vi "Configure Results Names.vi"(8 "error in":errorcluster, 11 "DAC ADV in":refnum<class "DAC ADV.lvclass">) -> (0 "error out":errorcluster, 3 "DAC ADV out":refnum<class "DAC ADV.lvclass">)   [LabVIEW 2019, in "DAC.lvlib" / "DAC ADV.lvclass"]
uses:
  DAC ADV.lvclass
  DAC ADV.lvclass/DAC ADV.ctl
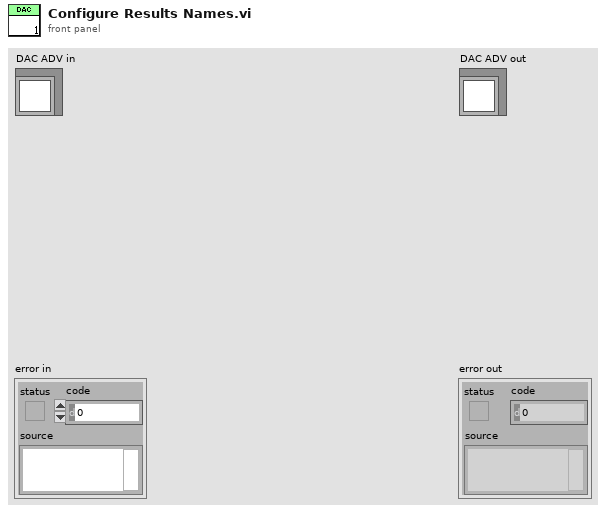
[diagram p1: front panel]
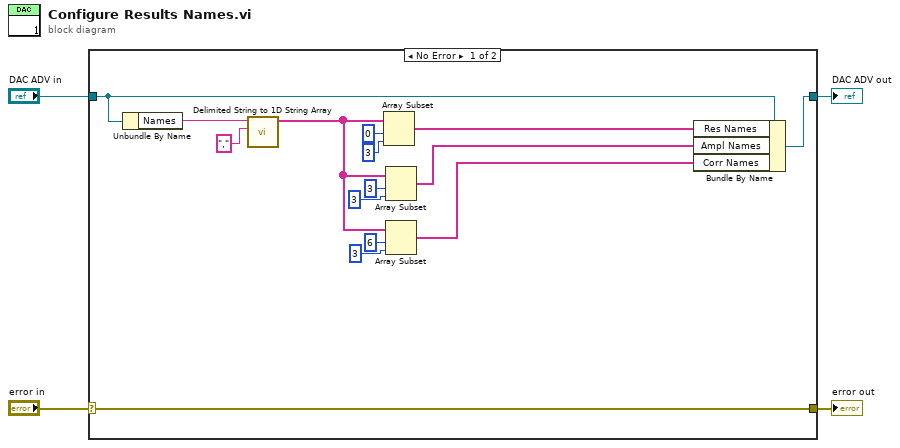
[diagram p0: block diagram]
diagram:
  n1 = case shown="No Error" "error in" {
    selector: "error in" -> [w19 w21]
    tunnel: [w19 w21] -> w3
    tunnel: [w18 w20] -> w1
    tunnel: "DAC ADV in" -> [w17 w20]
    frame No Error {
      n2 = Unbundle By Name(w17) -> ("Names"=w9:string)
      n3 = call <vilib>:"Delimited String to 1D String Array.vi"("delimiter"=",", "delimited string"=w9) -> ("string array"=w7:string[])  [unwired: 9 in]
      n4 = Array Subset(array=w7, index=0, length=3) -> (w8:string[])
      n5 = Array Subset(array=w7, index=3, length=3) -> (w6:string[])
      n6 = Array Subset(array=w7, index=6, length=3) -> (w5:string[])
      n7 = Bundle By Name(cluster=w17, "Res Names"=w8, "Ampl Names"=w6, "Corr Names"=w5) -> (w18:refnum<class "DAC ADV.lvclass">)
    }
    frame Error {
    }
  }
  "error out" <- w3
  "DAC ADV out" <- w1
